vi "Wheel of Doom State to Number of Power Cells.vi"(11 "Slot States":T1[](array[typedef])) -> (3 "Numeric":i32)   [LabVIEW 2019]
uses:
  Wheel of Doom Slot State.ctl
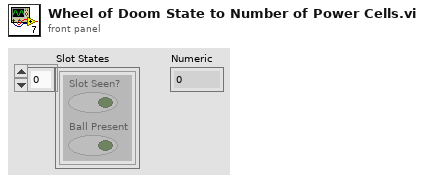
[diagram p1: front panel]
types:
  T1 = typedef "Wheel of Doom Slot State.ctl" = cluster{"Slot Seen?":bool, "Ball Present":bool}
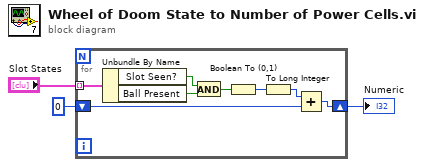
[diagram p0: block diagram]
diagram:
  n1 = for {
    tunnel: "Slot States" -> [w11] mode=indexing
    shift-right: [w5] -> w2
    shift-left: 0 -> [w4]
    n2 = Unbundle By Name(w11) -> ("Slot Seen?"=w9:bool, "Ball Present"=w10:bool)
    n3 = And(x=w9, y=w10) -> (x .and. y?=w8:bool)
    n4 = Boolean To (0,1)(Boolean=w8) -> (0, 1=w7:i16)
    n5 = To Long Integer(number=w7) -> (32bit integer=w6:i32)
    n6 = Add(x=w6, y=w4) -> (x+y=w5:i32)
  }
  "Numeric" <- w2
